vi "Set_speed_and_move.vi"() -> ()   [LabVIEW 2013]
panel:
  in  "Pulse Number 3":u32=10000 min=1 max=500000
  out "Command String 6":string="A:1+P10000"
  out "String Received 6":string="OK\r\n"
  out "Received String2 3":string="R\r\n"
  in  "Low Speed 3":u32=3000 min=1 max=500000
  in  "High Speed 3":u32=30000 min=1 max=500000
  in  "Acceleration Time 3":u16=100 max=1000
  out "Command String 5":string="D:1S3000F30000R100"
  out "String Received 5":string="OK\r\n"
  in  "Port Number Z":i8=8 min=0
  in  "Axis Number 3":u8=1
  out "OK speed 3":bool=TRUE
  out "OK move 3":bool=TRUE
  out "Received String2 2":string="R\r\n"
  out "String Received 4":string="OK\r\n"
  out "Command String 4":string="A:2+P10000"
  out "OK move 2":bool=TRUE
  in  "Pulse Number 2":u32=10000 min=1 max=500000
  in  "Axis Number 2":u8=2
  out "OK speed 2":bool=TRUE
  out "String Received 3":string="OK\r\n"
  out "Command String 3":string="D:2S1000F10000R100"
  in  "Acceleration Time 2":u16=100 max=1000
  in  "High Speed 2":u32=10000 min=1 max=500000
  in  "Low Speed 2":u32=1000 min=1 max=500000
  out "Received String2":string="R\r\n"
  out "String Received 2":string="OK\r\n"
  out "Command String 2":string="A:1+P10000"
  out "OK move 1":bool=TRUE
  in  "Pulse Number 1":u32=10000 min=1 max=500000
  in  "Axis Number 1":u8=1
  out "OK speed 1":bool=TRUE
  in  "Port Number":i8=7 min=0
  out "String Received":string="OK\r\n"
  out "Command String":string="D:1S1000F10000R100"
  in  "Acceleration Time":u16=100 max=1000
  in  "High Speed":u32=10000 min=1 max=500000
  in  "Low Speed":u32=1000 min=1 max=500000
  # "For tensile test (30 mm sample length):\nSet local origin as X (axis 1) 27000, Y (axis 2) 5000"
  # "Set speed"
  # "Move to the absolute position"
  # "Abs. position X\nin um"
  # "X"
  # "Abs. position Y\nin um"
  # "Y"
  # "Abs. position Z\nin um"
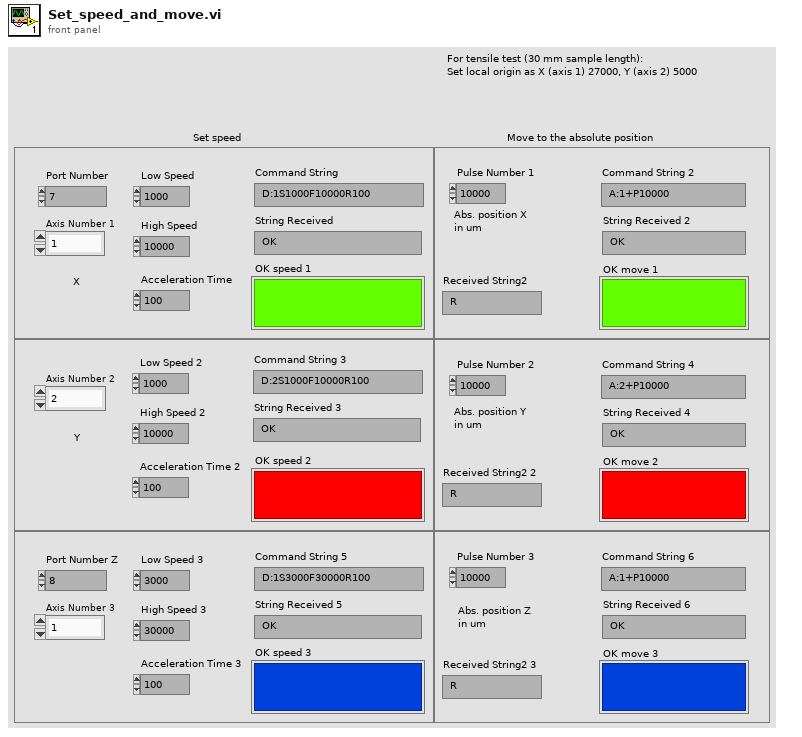
[diagram p1: front panel]
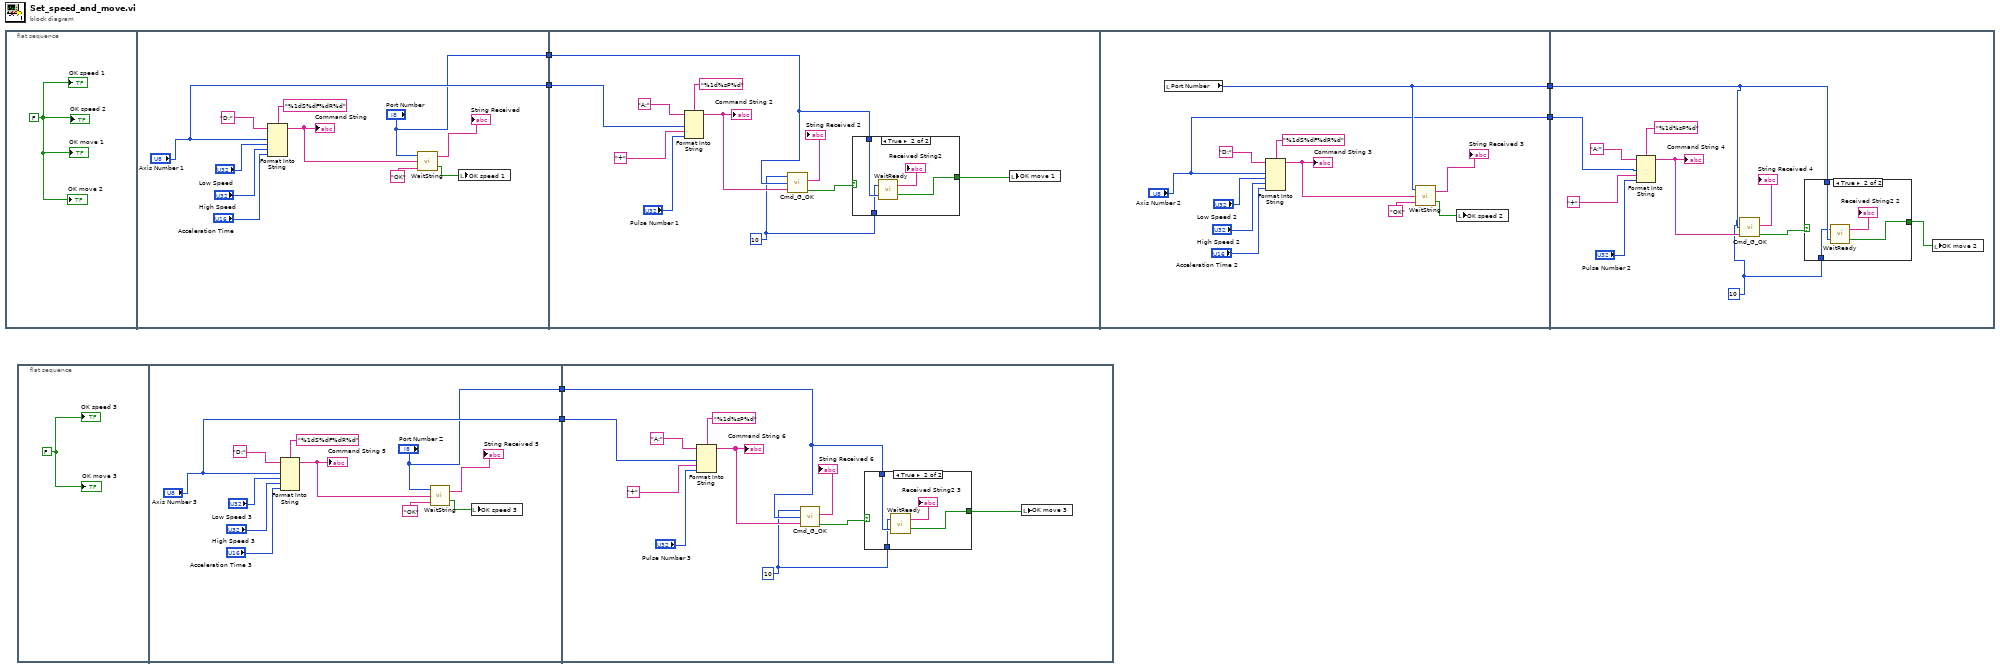
[diagram p0: block diagram]
diagram:
  n1 = flat-sequence {
    tunnel: ["Axis Number 1"] -> w6
    tunnel: ["Port Number"] -> w5
    tunnel: w6 -> [w22]
    tunnel: w5 -> [w21]
    tunnel: [w37] -> w4
    tunnel: ["Axis Number 2"] -> w3
    tunnel: w4 -> [w49]
    tunnel: w3 -> [w48]
    frame #0 {
      w7 = FALSE
      "OK speed 1" <- w7
      "OK speed 2" <- w7
      "OK move 1" <- w7
      "OK move 2" <- w7
    }
    frame #1 {
      n2 = Format Into String(format string="%1dS%dF%dR%d", initial string="D:", "Axis Number 1", "Low Speed", "High Speed", "Acceleration Time") -> (resulting string=w12:string)  [unwired: 1 in, 1 out]
      "Command String" <- w12
      n3 = call "WaitString.vi"("String to Receive"="OK", "String to Send"=w12, "PortNumber"="Port Number") -> ("OK Done"=w8:bool, "String Received"=→"String Received":string)
      n4 = local write "OK speed 1"(w8) -> ()
    }
    frame #2 {
      w19 = 10
      n5 = Format Into String(format string="%1d%sP%d", initial string="A:", w22, "+", "Pulse Number 1") -> (resulting string=w26:string)  [unwired: 1 in, 1 out]
      "Command String 2" <- w26
      n6 = call "Cmd_G_OK.vi"("Residence time"=w19, "PortNumber"=w21, "Command String"=w26) -> ("Received String2"=→"String Received 2":string, "OK Done"=w28:bool)  [unwired: 2 out]
      n7 = case shown="True" w28 {
        selector: w28 -> [w30 _]
        tunnel: w21 -> [_ w34]
        tunnel: [w30 w32] -> w20
        tunnel: w19 -> [_ w31]
        frame False {
        }
        frame True {
          n8 = call "WaitReady.vi"("PortNumber"=w34, "Residence time in ms"=w31) -> ("OK Done"=w32:bool, "String Received"=→"Received String2":string)
        }
      }
      n9 = local write "OK move 1"(w20) -> ()
    }
    frame #3 {
      n10 = local read "Port Number"() -> (w37:i8)
      n11 = Format Into String(format string="%1dS%dF%dR%d", initial string="D:", "Axis Number 2", "Low Speed 2", "High Speed 2", "Acceleration Time 2") -> (resulting string=w44:string)  [unwired: 1 in, 1 out]
      "Command String 3" <- w44
      n12 = call "WaitString.vi"("String to Receive"="OK", "String to Send"=w44, "PortNumber"=w37) -> ("OK Done"=w35:bool, "String Received"=→"String Received 3":string)
      n13 = local write "OK speed 2"(w35) -> ()
    }
    frame #4 {
      w46 = 10
      n14 = Format Into String(format string="%1d%sP%d", initial string="A:", w48, "+", "Pulse Number 2") -> (resulting string=w53:string)  [unwired: 1 in, 1 out]
      "Command String 4" <- w53
      n15 = call "Cmd_G_OK.vi"("Residence time"=w46, "PortNumber"=w49, "Command String"=w53) -> ("Received String2"=→"String Received 4":string, "OK Done"=w51:bool)  [unwired: 2 out]
      n16 = case shown="True" w51 {
        selector: w51 -> [w57 _]
        tunnel: [w57 w60] -> w47
        tunnel: w49 -> [_ w59]
        tunnel: w46 -> [_ w58]
        frame False {
        }
        frame True {
          n17 = call "WaitReady.vi"("PortNumber"=w59, "Residence time in ms"=w58) -> ("OK Done"=w60:bool, "String Received"=→"Received String2 2":string)
        }
      }
      n18 = local write "OK move 2"(w47) -> ()
    }
  }
  n19 = flat-sequence {
    tunnel: ["Axis Number 3"] -> w2
    tunnel: ["Port Number Z"] -> w1
    tunnel: w2 -> [w77]
    tunnel: w1 -> [w76]
    frame #0 {
      w62 = FALSE
      "OK speed 3" <- w62
      "OK move 3" <- w62
    }
    frame #1 {
      n20 = Format Into String(format string="%1dS%dF%dR%d", initial string="D:", "Axis Number 3", "Low Speed 3", "High Speed 3", "Acceleration Time 3") -> (resulting string=w67:string)  [unwired: 1 in, 1 out]
      "Command String 5" <- w67
      n21 = call "WaitString.vi"("String to Receive"="OK", "String to Send"=w67, "PortNumber"="Port Number Z") -> ("OK Done"=w63:bool, "String Received"=→"String Received 5":string)
      n22 = local write "OK speed 3"(w63) -> ()
    }
    frame #2 {
      w74 = 10
      n23 = Format Into String(format string="%1d%sP%d", initial string="A:", w77, "+", "Pulse Number 3") -> (resulting string=w81:string)  [unwired: 1 in, 1 out]
      "Command String 6" <- w81
      n24 = call "Cmd_G_OK.vi"("Residence time"=w74, "PortNumber"=w76, "Command String"=w81) -> ("Received String2"=→"String Received 6":string, "OK Done"=w83:bool)  [unwired: 2 out]
      n25 = case shown="True" w83 {
        selector: w83 -> [w85 _]
        tunnel: w76 -> [_ w89]
        tunnel: [w85 w87] -> w75
        tunnel: w74 -> [_ w86]
        frame False {
        }
        frame True {
          n26 = call "WaitReady.vi"("PortNumber"=w89, "Residence time in ms"=w86) -> ("OK Done"=w87:bool, "String Received"=→"Received String2 3":string)
        }
      }
      n27 = local write "OK move 3"(w75) -> ()
    }
  }
